vi "ProcessData.vi"(10 "Error Loacations":dbl[](array[numeric])=[332.0, 348.0, 364.0, 380.0], 11 "Read Info":T1[](array[typedef])=[{"Expected Value(s)"=[0], "Compare Locations"=[332, 340, 348, 356, 364, 372, 380, 388, 396]}, {"Expected Value(s)"=[170], "Compare Locations"=[540, 548, 556, 564, 572, 580, 588, 596, 604]}] {"Expected Value(s)" format="%.0x"}) -> (2 "Parity Error":bool, 3 "Read MIPI Data":cluster{"Read Data":u8[]}[](array[cluster])=[{"Read Data"=[170]}, {"Read Data"=[170]}] {"Read Data" format="%.0x"})   [LabVIEW 2013]
uses:
  Ctrls/ReadInfo.ctl
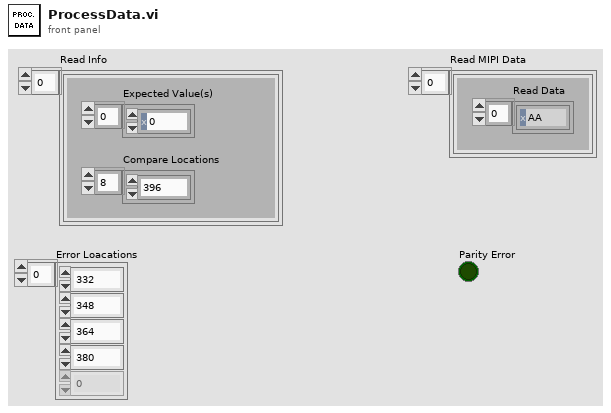
[diagram p1: front panel]
types:
  T1 = typedef "ReadInfo.ctl" = cluster{"Expected Value(s)":u8[], "Compare Locations":u32[]}
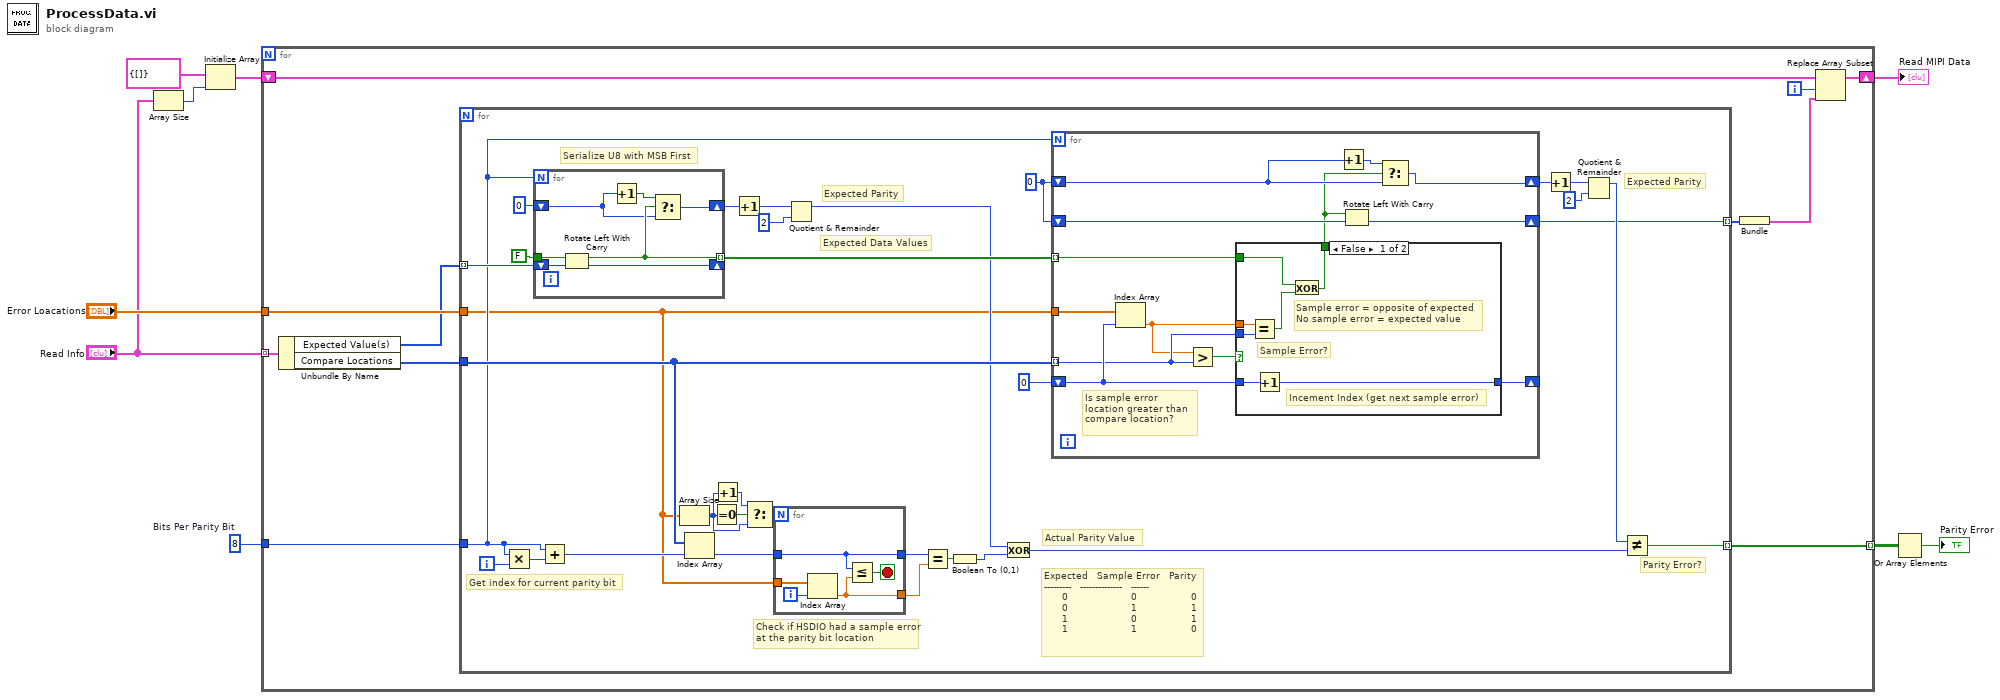
[diagram p0: block diagram]
diagram:
  w1 = 8  # Bits Per Parity Bit
  n1 = Array Size(array="Read Info") -> (size(s)=w6:i32)
  n2 = Initialize Array(cluster{u8[]} {[]} ("output cluster"), w6) -> (w8:cluster{u8[]}[])
  n3 = for {
    tunnel: "Error Loacations" -> [w20]
    tunnel: "Read Info" -> [w17] mode=indexing
    shift-right: [w15] -> w4
    shift-left: w8 -> [w14]
    tunnel: [w11] -> w3 mode=indexing
    tunnel: w1 -> [w10]
    i -> [w12]
    n4 = Unbundle By Name(w17) -> ("Expected Value(s)"=w18:u8[], "Compare Locations"=w19:u32[])
    n5 = for {
      tunnel: w20 -> [w26]
      tunnel: w19 -> [w52]
      tunnel: w18 -> [w42] mode=indexing
      tunnel: [w30] -> w16 mode=indexing
      tunnel: [w29] -> w11 mode=indexing
      tunnel: w10 -> [w28]
      i -> [w51]
      w43 = u8 0
      # "Serialize U8 with MSB First"
      # "Parity Error?"
      # "Expected   Sample Error   Parity\n---------   --------------   ------\n      0                     0                  0\n      0                     1                  1\n      1                     0                  1\n      1                     1                  0"
      # "Check if HSDIO had a sample error at the parity bit location"
      # "Get index for current parity bit"
      # "Expected Data Values"
      # "Expected Parity"
      # "Expected Parity"
      # "Actual Parity Value"
      n6 = Multiply(x=w28, y=w51) -> (x*y=w32:i32)
      n7 = for {
        N: w28 -> [_]
        shift-right: [w63] -> _
        shift-left: w42 -> [w64]
        tunnel: FALSE ("lsb carry out") -> [w62]
        tunnel: [w60] -> w40 mode=indexing
        shift-right: [w59] -> w36
        shift-left: u8 0 -> [w58]
        n8 = Rotate Left With Carry(2:w64, 3:w62) -> (0:w63:u8, 1:w60:bool)
        n9 = Increment(x=w58) -> (x+1=w61:u8)
        n10 = Select(t=w61, s=w60, f=w58) -> (s? t:f=w59:u8)
      }
      n11 = Add(x=w28, y=w32) -> (x+y=w31:i32)
      n12 = Array Size(array=w26) -> (size(s)=w22:i32)
      n13 = Index Array(array=w52, index=w31) -> (element=w50:u32)
      n14 = Equal To 0?(x=w22) -> (x = 0?=w24:bool)
      n15 = Increment(x=w22) -> (x+1=w23:i32)
      n16 = Increment(x=w36) -> (x+1=w38:u8)
      n17 = Select(t=w23, s=w24, f=w22) -> (s? t:f=w21:i32)
      n18 = for {
        N: w21 -> [_]
        tunnel: w50 -> [w57]
        tunnel: w26 -> [w55]
        tunnel: [w54] -> w48
        tunnel: [w57] -> w49
        i -> [w53]
        stop <- w56 stop-if-true
        n19 = Index Array(array=w55, index=w53) -> (element=w54:dbl)
        n20 = Less Or Equal?(x=w57, y=w54) -> (x <= y?=w56:bool)
      }
      n21 = Quotient & Remainder(x=w38, y=u8 2) -> (x-y*floor(x/y)=w34:u8)  [unwired: 1 out]
      n22 = Equal?(x=w49, y=w48) -> (x = y?=w47:bool)
      n23 = Boolean To (0,1)(Boolean=w47) -> (0, 1=w35:i16)
      n24 = Exclusive Or(1:w35, 2:w34) -> (0:w33:i16)
      n25 = for {
        N: w28 -> [_]
        tunnel: w26 -> [w77]
        tunnel: w52 -> [w72] mode=indexing
        shift-right: [w76] -> _
        shift-left: 0 -> [w75]
        shift-right: [w74] -> w30
        shift-left: w43 -> [w73]
        shift-right: [w71] -> w27
        shift-left: w43 -> [w70]
        tunnel: w40 -> [w69] mode=indexing
        # "Is sample error location greater than compare location?"
        n26 = Index Array(array=w77, index=w75) -> (element=w66:dbl)
        n27 = Greater?(x=w66, y=w72) -> (0:w65:bool)
        n28 = case shown="False" w65 {
          tunnel: [w84 w86] -> w76
          tunnel: w75 -> [w83 w86]
          tunnel: w66 -> [w82 _]
          tunnel: w72 -> [w81 _]
          tunnel: w69 -> [w80 w85]
          tunnel: [w78 w85] -> w67
          frame False {
            # "Sample error = opposite of expected\nNo sample error = expected value"
            # "Incement Index (get next sample error)"
            # "Sample Error?"
            n29 = Equal?(x=w82, y=w81) -> (x = y?=w79:bool)
            n30 = Increment(x=w83) -> (x+1=w84:i32)
            n31 = Exclusive Or(1:w79, 2:w80) -> (0:w78:bool)
          }
          frame True {
            # "Keep same index for next compare location"
            # "Sample Error Location Greater"
          }
        }
        n32 = Increment(x=w70) -> (x+1=w68:u8)
        n33 = Rotate Left With Carry(2:w73, 3:w67) -> (0:w74:u8)  [unwired: 1 out]
        n34 = Select(t=w68, s=w67, f=w70) -> (s? t:f=w71:u8)
      }
      n35 = Increment(x=w27) -> (x+1=w25:u8)
      n36 = Quotient & Remainder(x=w25, y=u8 2) -> (x-y*floor(x/y)=w46:u8)  [unwired: 1 out]
      n37 = Not Equal?(x=w46, y=w33) -> (x != y?=w29:bool)
    }
    n38 = Bundle(w16) -> (w13:cluster{u8[]})  [unwired: 1 in]
    n39 = Replace Array Subset(array=w14, new element=w13, index=w12) -> (w15:cluster{u8[]}[])
  }
  "Read MIPI Data" <- w4
  n40 = Or Array Elements(Boolean array=w3) -> (logical OR=→"Parity Error":bool)
